vi "real-time-fault-handler.vi"() -> ()   [LabVIEW 2018]
uses:
  <vilib>/Platform/TimedLoop/XDataNode/timing_clust.ctl
  <vilib>/Platform/TimedLoop/XDataNode/nitl_modes.ctl
  <vilib>/Platform/TimedLoop/XDataNode/wakeup.ctl
  <vilib>/rvi/Emulation/niFpgaSctlEmulationGetInTimedLoop.vi
  <vilib>/rvi/Emulation/niFpgaEmulationReportErrorSimple.vi
  <vilib>/rvi/Emulation/niFpgaGetClockAttributes.vi
  <vilib>/rvi/Emulation/niFpgaCriticalErrorInLSC.vi
  <vilib>/rvi/eio/common/nirviEmuTemplateMethod_errors.vi
  <vilib>/platform/TimedLoop/XDataNode/XDataNode.xnode
  <vilib>/eio/EIONode/EIONode.xnode
  <vilib>/Platform/TimedLoop/XDataNode/XDNodeRunTimeDep.lvlib
panel:
  out "x > y?":bool
  in  "y":bool
  in  "stop":bool
  out "Numeric 2":u32
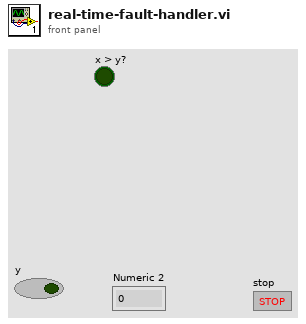
[diagram p1: front panel]
types:
  T1 = typedef "XDNodeRunTimeDep.lvlib/timing_clust.ctl" = cluster{"Expected End [f-1]":u64, "Actual End [f-1]":u64, "Finished Late? [f-1]":bool, "Expected End [i-1]":u64, "Actual End [i-1]":u64, "Finished Late? [i-1]":bool, "Expected Start [i]":u64, "Actual Start [i]":u64, "Expected Start [f]":u64, "Actual Start [f]":u64, "Source Name":string, "Structure Name":string, "Period":i64, "Deadline":i64, "Offset":i64, "Start":i64, "Priority":i32, "Timeout":i32, "Mode":T2, "Wakeup Reason":T3, "Error":errorcluster, "Source Type":string, "Secondary Source Type":string, "Global End Time":u64, "Global Start Time":u64, "Frame Duration":u64, "Iteration Duration":u64, "Assigned CPU":i32, "I/O Scan Engine Mode":u32}
  T2 = typedef "XDNodeRunTimeDep.lvlib/nitl_modes.ctl" = enum32{"No Change", "Process missed periods, maintain original phase", "Discard missed periods, maintain original phase", "Process missed periods, ignore original phase", "Discard missed periods, ignore original phase"}
  T3 = typedef "XDNodeRunTimeDep.lvlib/wakeup.ctl" = enum32{"Normal", "Aborted", "Asynchronous wakeup", "Timing source error", "Timed loop error", "Timeout"}
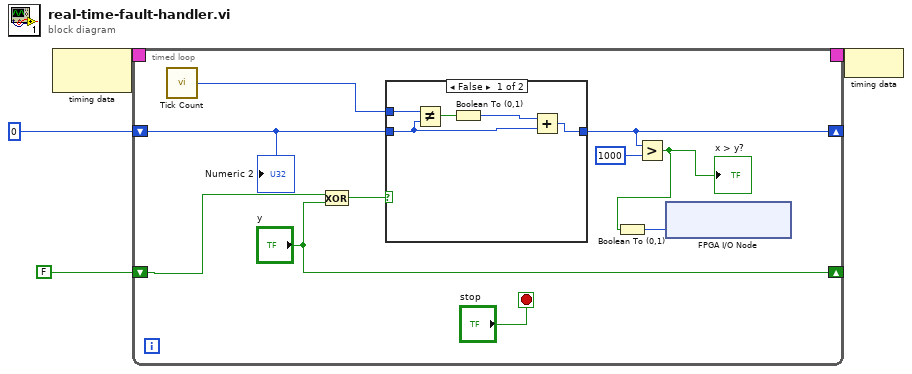
[diagram p0: block diagram]
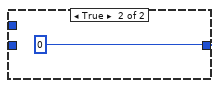
[diagram p2: hidden frame]
diagram:
  n1 = node-c288() -> (w4:T1)  [unwired: 1 in]
  n2 = timed-loop {
    timing: w4 -> [_]
    timing-out: [_] -> w3
    shift-right: ["y"] -> _
    shift-left: FALSE -> [w10]
    shift-right: [w8] -> _
    shift-left: u32 0 ("Numeric") -> [w14]
    stop <- "stop" stop-if-true
    n3 = call "Tick Count"() -> ("Tick Count(mSec)"=w13:u8)
    n4 = Exclusive Or(1:"y", 2:w10) -> (0:w11:bool)
    n5 = case shown="False" w11 {
      tunnel: w14 -> [w16 _]
      tunnel: [w15 u8 0 ("Numeric")] -> w8
      tunnel: w13 -> [w17 _]
      frame False {
        n6 = Not Equal?(x=w17, y=w16) -> (x != y?=w19:bool)
        n7 = Boolean To (0,1)(Boolean=w19) -> (0, 1=w18:i16)
        n8 = Add(x=w18, y=w16) -> (x+y=w15:u32)
      }
      frame True {
      }
    }
    n9 = Greater?(x=w8, y=i16 1000) -> (0:w5:bool)
    "x > y?" <- w5
    n10 = Boolean To (0,1)(Boolean=w5) -> (0, 1=w6:i16)
    n11 = xnode "FPGA I/O Node"("USER FPGA LED"=w6) -> ()  [unwired: 1 in, 1 out]
    "Numeric 2" <- w14
  }
  n12 = node-c288(w3) -> ()
